vi "eStopShared.vi"(7 "Command":T1=enum."Get E-Stop", 8 "Error In":errorcluster, 11 "E-Stop":bool) -> (0 "Error Out":errorcluster, 3 "E-Stop Out":bool)   [LabVIEW 2011]
uses:
  2 Typedefs/eStopCommand.ctl
  2 Globals/2 Global.vi
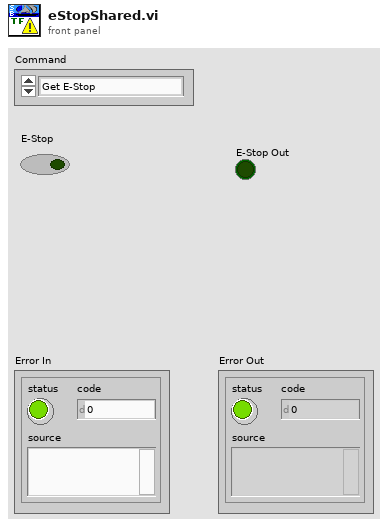
[diagram p1: front panel]
types:
  T1 = typedef "eStopCommand.ctl" = enum16{"Reset E-Stop", "Get E-Stop", "Set E-Stop"}
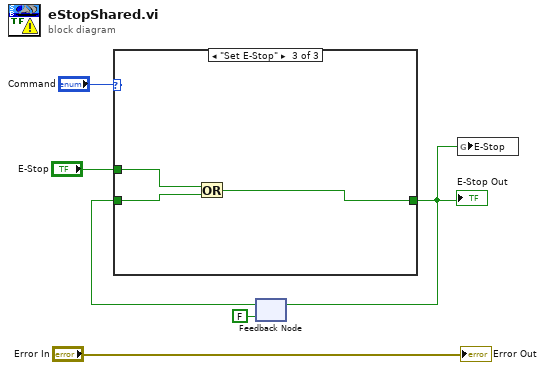
[diagram p0: block diagram]
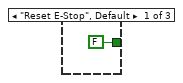
[diagram p2: hidden frame]
diagram:
  n1 = feedback #1(FALSE) -> (w2:bool)
  n2 = case shown="\"Set E-Stop\"" "Command" {
    tunnel: "E-Stop" -> [_ _ w11]
    tunnel: w2 -> [_ w8 w10]
    tunnel: [FALSE w8 w9] -> w1
    frame "Reset E-Stop", Default {
    }
    frame "Get E-Stop" {
    }
    frame "Set E-Stop" {
      n3 = Or(x=w11, y=w10) -> (x .or. y?=w9:bool)
    }
  }
  "E-Stop Out" <- w1
  n4 = feedback-in #1(w1) -> ()
  n5 = global write "2 Global.vi" "E-Stop"(w1) -> ()
  "Error Out" <- "Error In"
